vi "Get Fit Settings.vi"(6 "Fit Model":T2, 8 "Error In":errorcluster, 9 "Additional Parameters":variant, 10 "Fixed Parameters":T1, 11 "XY Graph Ref":refnum<vi>) -> (0 "Error Out":errorcluster, 2 "Additional Fit Settings":variant, 3 "LM Function & Gradient":refnum<vi>)   [LabVIEW 2019]
uses:
  Fit Models.ctl
  D-Only Fixed Parameters.ctl
  N Components Additional Fit Settings.ctl
  Variant to Data.lvlib
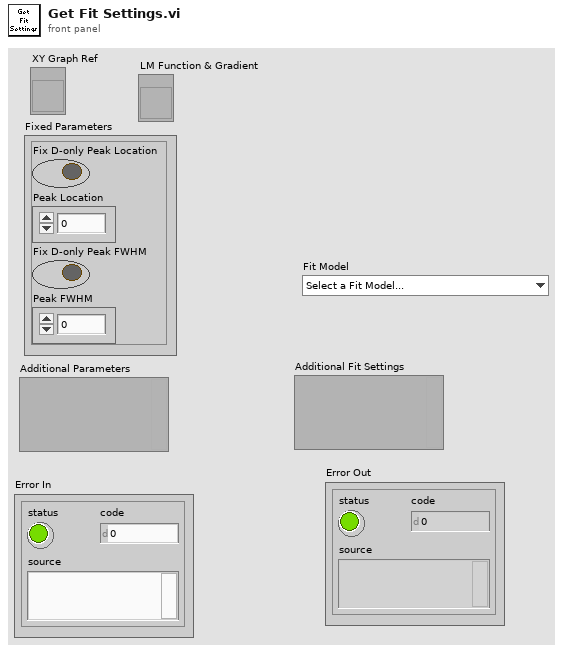
[diagram p1: front panel]
types:
  T1 = typedef "D-Only Fixed Parameters.ctl" = cluster{"Fix D-only Peak Location":bool, "Peak Location":dbl, "Fix D-only Peak FWHM":bool, "Peak FWHM":dbl}
  T2 = typedef "Fit Models.ctl" = enum16{"Select a Fit Model...", "           Single Peak", "Gaussian", "Asymmetric Gaussian", "Lorentzian", "Asymmetric Lorentzian", "Gaussian/Lorentzian", "Lorentzian/Gaussian", "           Double Peak", "Two Gaussians", "Two Asymmetric Gaussians", "Two H-Connected Gaussians", "Two T-Connected Gaussians", "Two H-Connected Asymmetric Gaussians", "Two T-Connected Asymmetric Gaussians", "           Triple Peak", "Three Gaussians", "Three Asymmetric Gaussians", "              Decays", "Single Exponential", "Two Exponentials", "               ACF", "2D Gaussian ACF", "2D Gaussian + Blinking ACF", "2D Gaussian + Flow ACF", "3D Gaussian ACF", "3D Gaussian + Blinking ACF", "             Multiplot", "2D Gaussian ACF & 2D Gaussian + Flow ACF"}
  T3 = typedef "N Components Additional Fit Settings.ctl" = cluster{"Fixed Parameters":T1, "Cursor Coordinates":dbl[], "Data Split Point":i32}
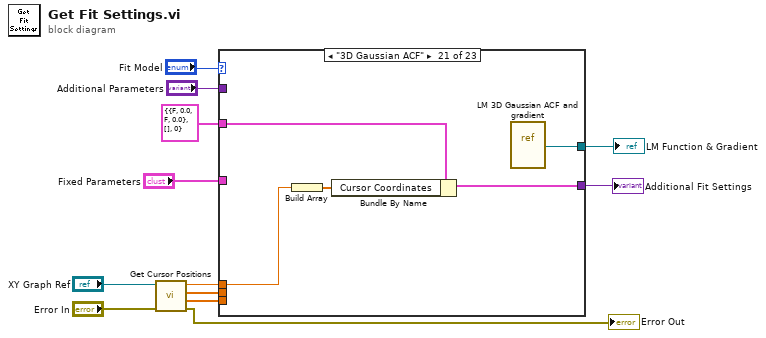
[diagram p0: block diagram]
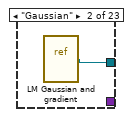
[diagram p3: hidden frame]
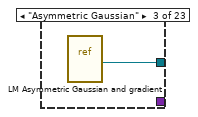
[diagram p4: hidden frame]
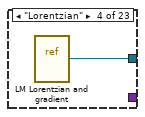
[diagram p5: hidden frame]
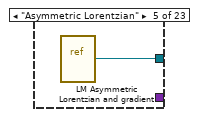
[diagram p6: hidden frame]
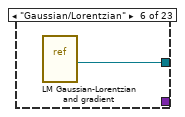
[diagram p7: hidden frame]
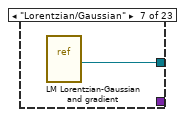
[diagram p8: hidden frame]
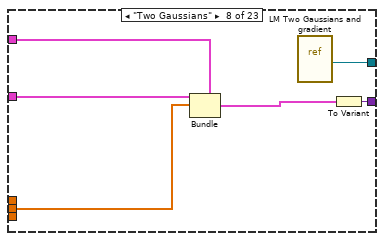
[diagram p9: hidden frame]
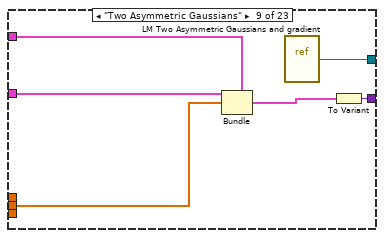
[diagram p10: hidden frame]
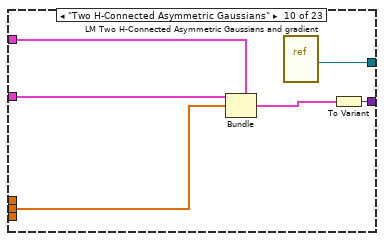
[diagram p11: hidden frame]
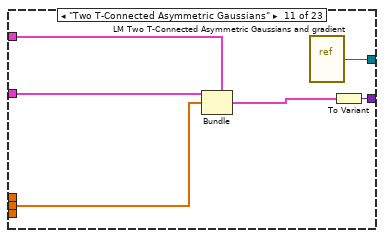
[diagram p12: hidden frame]
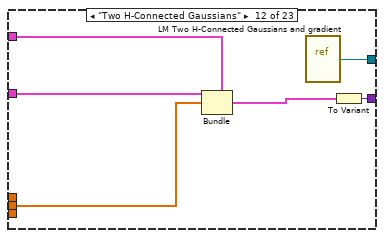
[diagram p13: hidden frame]
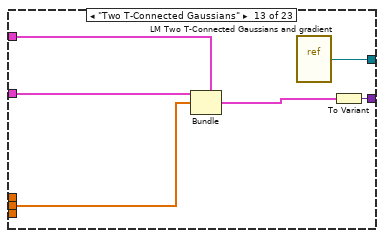
[diagram p14: hidden frame]
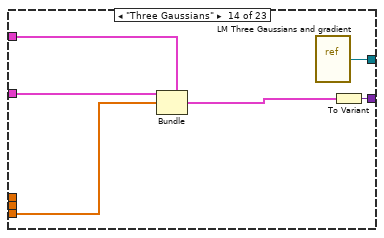
[diagram p15: hidden frame]
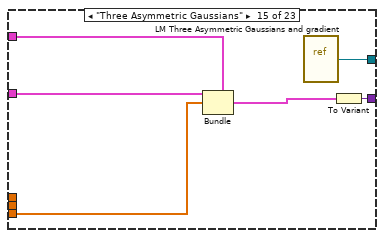
[diagram p16: hidden frame]
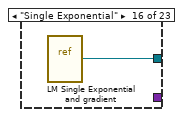
[diagram p17: hidden frame]
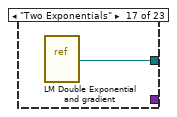
[diagram p18: hidden frame]
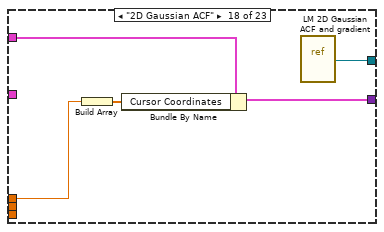
[diagram p19: hidden frame]
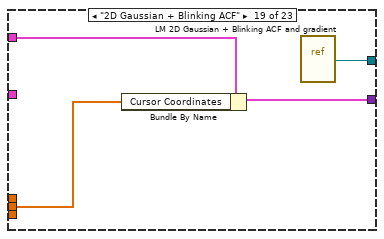
[diagram p20: hidden frame]
diagram:
  n1 = call "Get Cursor Positions.vi"("Error In"="Error In", "XYGraph in"="XY Graph Ref") -> ("Error Out"=→"Error Out":errorcluster, "Cursor 1-3 Positions"=w5:dbl[], "Cursor 1 & 2 Positions"=w6:dbl[], "Cursor 1 Position"=w7:dbl)  [unwired: 6 in]
  n2 = case shown="\"3D Gaussian ACF\"" "Fit Model" {
    tunnel: "Fixed Parameters" -> [_ _ _ _ _ _ _ w24 w30 w36 w42 w48 w54 w60 w66 _ _ _ _ _ _ _ _]
    tunnel: [_ _ _ _ _ _ _ w22 w28 w34 w40 w46 w52 w58 w64 _ _ w70 w76 w80 w83 w89 w94] -> w11
    tunnel: [_ w13 w14 w15 w16 w17 w18 w21 w27 w32 w38 w45 w50 w57 w63 w67 w68 w73 w77 w81 w86 w90 w96] -> w8
    tunnel: w5 -> [_ _ _ _ _ _ _ _ _ _ _ _ _ w56 w62 _ _ _ _ _ _ _ _]
    tunnel: w6 -> [_ _ _ _ _ _ _ w20 w26 w33 w39 w44 w51 _ _ _ _ _ w75 w79 _ w88 w91]
    tunnel: w7 -> [_ _ _ _ _ _ _ _ _ _ _ _ _ _ _ _ _ w72 _ _ w85 _ _]
    tunnel: T3 {"Fixed Parameters"={"Fix D-only Peak Location"=FALSE, "Peak Location"=0.0, "Fix D-only Peak FWHM"=FALSE, "Peak FWHM"=0.0}, "Cursor Coordinates"=[], "Data Split Point"=0} ("N Components Additional Fit Settings") -> [_ _ _ _ _ _ _ w19 w25 w31 w37 w43 w49 w55 w61 _ _ w69 w74 w78 w82 w87 w95]
    tunnel: "Additional Parameters" -> [_ _ _ _ _ _ _ _ _ _ _ _ _ _ _ _ _ _ _ _ _ _ w93]
    frame "Select a Fit Model...", Default {
    }
    frame "Gaussian" {
      n3 = vi-ref "LM Gaussian and gradient.vi"() -> (w13:refnum<vi>)
    }
    frame "Asymmetric Gaussian" {
      n4 = vi-ref "LM Asymmetric Gaussian and gradient.vi"() -> (w14:refnum<vi>)
    }
    frame "Lorentzian" {
      n5 = vi-ref "LM Lorentzian and gradient.vi"() -> (w15:refnum<vi>)
    }
    frame "Asymmetric Lorentzian" {
      n6 = vi-ref "LM Asymmetric Lorentzian and gradient.vi"() -> (w16:refnum<vi>)
    }
    frame "Gaussian/Lorentzian" {
      n7 = vi-ref "LM Gaussian-Lorentzian and gradient.vi"() -> (w17:refnum<vi>)
    }
    frame "Lorentzian/Gaussian" {
      n8 = vi-ref "LM Lorentzian-Gaussian and gradient.vi"() -> (w18:refnum<vi>)
    }
    frame "Two Gaussians" {
      n9 = Bundle(cluster=w19, "Fixed Parameters"=w24, "Cursor Coordinates"=w20) -> (w23:T3)  [unwired: 1 in]
      n10 = vi-ref "LM Two Gaussians and gradient.vi"() -> (w21:refnum<vi>)
      n11 = To Variant(anything=w23) -> (Variant=w22:variant)
    }
    frame "Two Asymmetric Gaussians" {
      n12 = Bundle(cluster=w25, "Fixed Parameters"=w30, "Cursor Coordinates"=w26) -> (w29:T3)  [unwired: 1 in]
      n13 = vi-ref "LM Two Asymmetric Gaussians and gradient.vi"() -> (w27:refnum<vi>)
      n14 = To Variant(anything=w29) -> (Variant=w28:variant)
    }
    frame "Two H-Connected Asymmetric Gaussians" {
      n15 = Bundle(cluster=w31, "Fixed Parameters"=w36, "Cursor Coordinates"=w33) -> (w35:T3)  [unwired: 1 in]
      n16 = vi-ref "LM Two H-Connected Asymmetric Gaussians and gradient.vi"() -> (w32:refnum<vi>)
      n17 = To Variant(anything=w35) -> (Variant=w34:variant)
    }
    frame "Two T-Connected Asymmetric Gaussians" {
      n18 = Bundle(cluster=w37, "Fixed Parameters"=w42, "Cursor Coordinates"=w39) -> (w41:T3)  [unwired: 1 in]
      n19 = vi-ref "LM Two T-Connected Asymmetric Gaussians and gradient.vi"() -> (w38:refnum<vi>)
      n20 = To Variant(anything=w41) -> (Variant=w40:variant)
    }
    frame "Two H-Connected Gaussians" {
      n21 = Bundle(cluster=w43, "Fixed Parameters"=w48, "Cursor Coordinates"=w44) -> (w47:T3)  [unwired: 1 in]
      n22 = vi-ref "LM Two H-Connected Gaussians and gradient.vi"() -> (w45:refnum<vi>)
      n23 = To Variant(anything=w47) -> (Variant=w46:variant)
    }
    frame "Two T-Connected Gaussians" {
      n24 = Bundle(cluster=w49, "Fixed Parameters"=w54, "Cursor Coordinates"=w51) -> (w53:T3)  [unwired: 1 in]
      n25 = vi-ref "LM Two T-Connected Gaussians and gradient.vi"() -> (w50:refnum<vi>)
      n26 = To Variant(anything=w53) -> (Variant=w52:variant)
    }
    frame "Three Gaussians" {
      n27 = Bundle(cluster=w55, "Fixed Parameters"=w60, "Cursor Coordinates"=w56) -> (w59:T3)  [unwired: 1 in]
      n28 = vi-ref "LM Three Gaussians and gradient.vi"() -> (w57:refnum<vi>)
      n29 = To Variant(anything=w59) -> (Variant=w58:variant)
    }
    frame "Three Asymmetric Gaussians" {
      n30 = Bundle(cluster=w61, "Fixed Parameters"=w66, "Cursor Coordinates"=w62) -> (w65:T3)  [unwired: 1 in]
      n31 = vi-ref "LM Three Asymmetric Gaussians and gradient.vi"() -> (w63:refnum<vi>)
      n32 = To Variant(anything=w65) -> (Variant=w64:variant)
    }
    frame "Single Exponential" {
      n33 = vi-ref "LM Single Exponential and gradient.vi"() -> (w67:refnum<vi>)
    }
    frame "Two Exponentials" {
      n34 = vi-ref "LM Double Exponential and gradient.vi"() -> (w68:refnum<vi>)
    }
    frame "2D Gaussian ACF" {
      n35 = Build Array(w72) -> (w71:dbl[])
      n36 = Bundle By Name(cluster=w69, "Cursor Coordinates"=w71) -> (w70:T3)
      n37 = vi-ref "LM 2D Gaussian ACF and gradient.vi"() -> (w73:refnum<vi>)
    }
    frame "2D Gaussian + Blinking ACF" {
      n38 = Bundle By Name(cluster=w74, "Cursor Coordinates"=w75) -> (w76:T3)
      n39 = vi-ref "LM 2D Gaussian + Blinking ACF and gradient.vi"() -> (w77:refnum<vi>)
    }
    frame "2D Gaussian + Flow ACF" {
      n40 = Bundle By Name(cluster=w78, "Cursor Coordinates"=w79) -> (w80:T3)
      n41 = vi-ref "LM 2D Gaussian + Flow ACF and gradient.vi"() -> (w81:refnum<vi>)
    }
    frame "3D Gaussian ACF" {
      n42 = Build Array(w85) -> (w84:dbl[])
      n43 = Bundle By Name(cluster=w82, "Cursor Coordinates"=w84) -> (w83:T3)
      n44 = vi-ref "LM 3D Gaussian ACF and gradient.vi"() -> (w86:refnum<vi>)
    }
    frame "3D Gaussian + Blinking ACF" {
      n45 = Bundle By Name(cluster=w87, "Cursor Coordinates"=w88) -> (w89:T3)
      n46 = vi-ref "LM 3D Gaussian + Blinking ACF and gradient.vi"() -> (w90:refnum<vi>)
    }
    frame "2D Gaussian ACF & 2D Gaussian + Flow ACF" {
      n47 = call "Variant to I32.vi"("Variant"=w93) -> ("Value"=w92:i32)  [unwired: 8 in]
      n48 = Bundle By Name(cluster=w95, "Data Split Point"=w92, "Cursor Coordinates"=w91) -> (w94:T3)
      n49 = vi-ref "LM 2D Gaussian ACF + Flow and gradient (Global).vi"() -> (w96:refnum<vi>)
    }
  }
  "Additional Fit Settings" <- w11
  "LM Function & Gradient" <- w8
